vi "Arduino Error.vi"(8 "error in":errorcluster, 10 "Reply":string) -> (0 "error out":errorcluster)   [LabVIEW 2023, in "Arduino DAQ.lvlib"]
uses:
  Arduino DAQ.lvlib
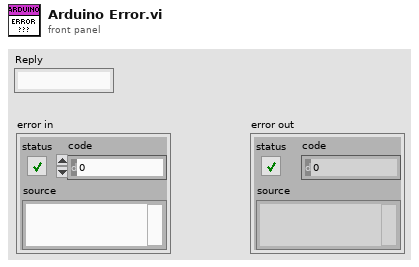
[diagram p1: front panel]
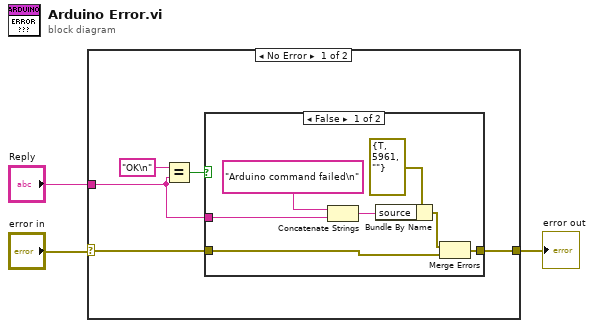
[diagram p0: block diagram]
diagram:
  n1 = case shown="No Error" "error in" {
    selector: "error in" -> [w5 w17]
    tunnel: "Reply" -> [w4 _]
    tunnel: [w6 w17] -> w2
    frame No Error {
      n2 = Equal?(x="OK\n" ("y"), y=w4) -> (x = y?=w7:bool)
      n3 = case shown="False" w7 {
        tunnel: [w15 w16] -> w6
        tunnel: w5 -> [w14 w16]
        tunnel: w4 -> [w10 _]
        frame False {
          n4 = Concatenate Strings("Arduino command failed\n" ("string"), w10) -> (w11:string)
          n5 = Bundle By Name(cluster=errorcluster {"status"=TRUE, "code"=5961, "source"=""} ("error constant"), "source"=w11) -> (w12:errorcluster)
          n6 = Merge Errors(w12, w14) -> (w15:errorcluster)
        }
        frame True {
        }
      }
    }
    frame Error {
    }
  }
  "error out" <- w2
